vi "Write Path.vi"(8 "error in":errorcluster, 10 "Path":path, 11 "Config in":refnum<class "Config.lvclass">) -> (0 "error out":errorcluster, 3 "Config out":refnum<class "Config.lvclass">)   [LabVIEW 2023, in "Config.lvlib" / "Config.lvclass"]
uses:
  Config.lvclass
  Config.lvclass/Config.ctl
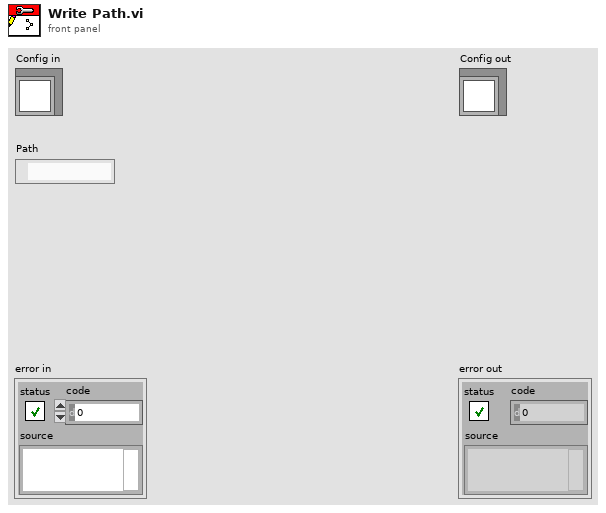
[diagram p1: front panel]
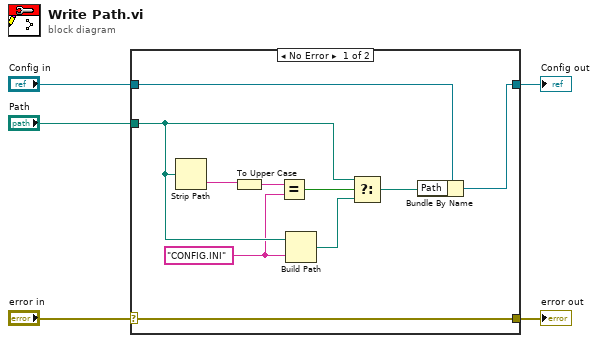
[diagram p0: block diagram]
diagram:
  n1 = case shown="No Error" "error in" {
    selector: "error in" -> [w15 w16]
    tunnel: [w15 w16] -> w4
    tunnel: [w13 w17] -> w2
    tunnel: "Config in" -> [w14 w17]
    tunnel: "Path" -> [w8 _]
    frame No Error {
      w7 = "CONFIG.INI" ("y")
      n2 = Strip Path(path=w8) -> (name=w12:string)  [unwired: 1 out]
      n3 = To Upper Case(1:w12) -> (0:w11:string)
      n4 = Equal?(x=w11, y=w7) -> (x = y?=w10:bool)
      n5 = Build Path(base path=w8, name or relative path=w7) -> (appended path=w6:path)
      n6 = Select(t=w8, s=w10, f=w6) -> (s? t:f=w9:path)
      n7 = Bundle By Name(cluster=w14, "Path"=w9) -> (w13:refnum<class "Config.lvclass">)
    }
    frame Error {
    }
  }
  "error out" <- w4
  "Config out" <- w2
